vi "GT Ln XYZAG0Override2.vi"(0 "cardNum":i16, 1 "z":i32, 2 "synVel":dbl, 3 "fifo":i16, 5 "crd":i16, 7 "x":i32, 9 "y":i32, 11 "error in (no error)":errorcluster caption="错误输入（无错误）", 12 "a":i32, 13 "synAcc":dbl) -> (4 "function return":i16, 15 "error out":errorcluster caption="错误输出")   [LabVIEW 2014, in "gts.lvlib"]
doc: "GT_API GT_LnXYZAG0Override2(short cardNum,short crd,long x,long y,long z,long a,double synVel,double synAcc,short fifo=0);"
uses:
  gts.lvlib
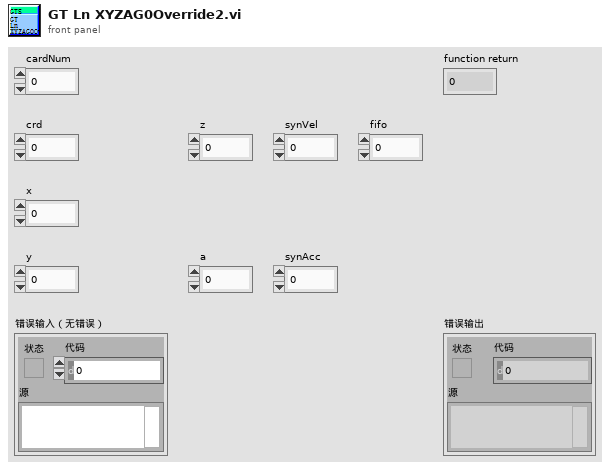
[diagram p1: front panel]
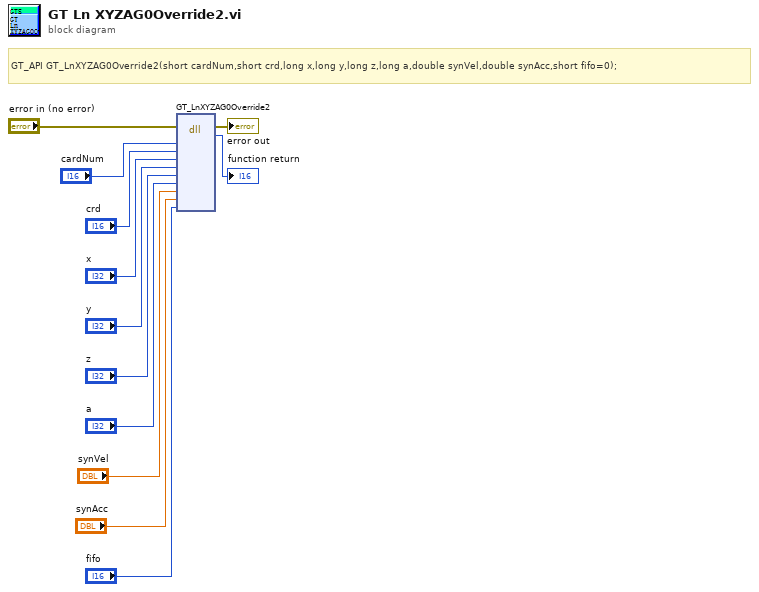
[diagram p0: block diagram]
diagram:
  # "GT_API GT_LnXYZAG0Override2(short cardNum,short crd,long x,long y,long z,long a,double synVel,double synAcc,short fifo=0);"
  n1 = dll-call lib="PTH2habs D固高科技资料GTS控制卡GTS卡18年上半年资料dllVC32bit\nmulti_cardgts.*" fn="GT_LnXYZAG0Override2"(error in="error in (no error)", "cardNum"="cardNum", "crd"="crd", "x"="x", "y"="y", "z"="z", "a"="a", "synVel"="synVel", "synAcc"="synAcc", "fifo"="fifo") -> (error out=→"error out":errorcluster, →"function return":i16)  [unwired: 11 in, 1 out]
